vi "Full Code using SensorDAQ.vi"() -> ()   [LabVIEW 2012]
uses:
  <vilib>/Utility/file.llb/Write To Spreadsheet File (string).vi
  <vilib>/express/express arith-compare/Formula/XNode/ExpressFormulaBlockNode.xnode
panel:
  in  "?":bool
  out "Nitrogen Compounds \n(NOx)  ppm":dbl(graph)
  out "Chlorine Gas (Cl2)  ppm":dbl(graph)
  out "Ozone (O3) ppm":dbl(graph)
  out "Nitrogen Compounds \n(NOx)  ppm_percentage":dbl
  out "Chlorine Gas (Cl2)  ppm_percentage":dbl
  out "Ozone (O3) ppm_percentage":dbl
  out "Nitrogen Compounds \n(NOx)  ppm":dbl
  out "Chlorine Gas (Cl2)  ppm":dbl
  out "Ozone (O3) ppm":dbl
  in  "Ro for MQ131":dbl
  out "Methane (CH4)  ppm":dbl(graph)
  out "Carbon Monoxide (CO)  ppm":dbl(graph)
  out "Butane (LPG) ppm":dbl(graph)
  out "Methane (CH4)\nppm_percentage":dbl
  out "Carbon Monoxide (CO)  ppm_percentage":dbl
  out "Butane (LPG) ppm_percentage":dbl
  out "Methane (CH4)  ppm":dbl
  out "Carbon Monoxide (CO)  ppm":dbl
  out "Butane   (LPG) ppm":dbl
  in  "Ro for MQ9":dbl
  out "CH 3 PH":dbl caption="CH 3 Auto-ID"
  out "CH 2 Conductivity":dbl caption="CH 2 Auto-ID"
  out "CH 1 Temperature":dbl caption="CH 1 Auto-ID"
  in  "file path (use dialog)":path
  out "Raw Voltage MQ9 Gas Sensor":dbl
  out "Raw Voltage MQ131 Ozone Sensor":dbl
  # "Vernier Sensors"
  # "MQ9 Gas Sensor"
  # "MQ131 Ozone Sensor"
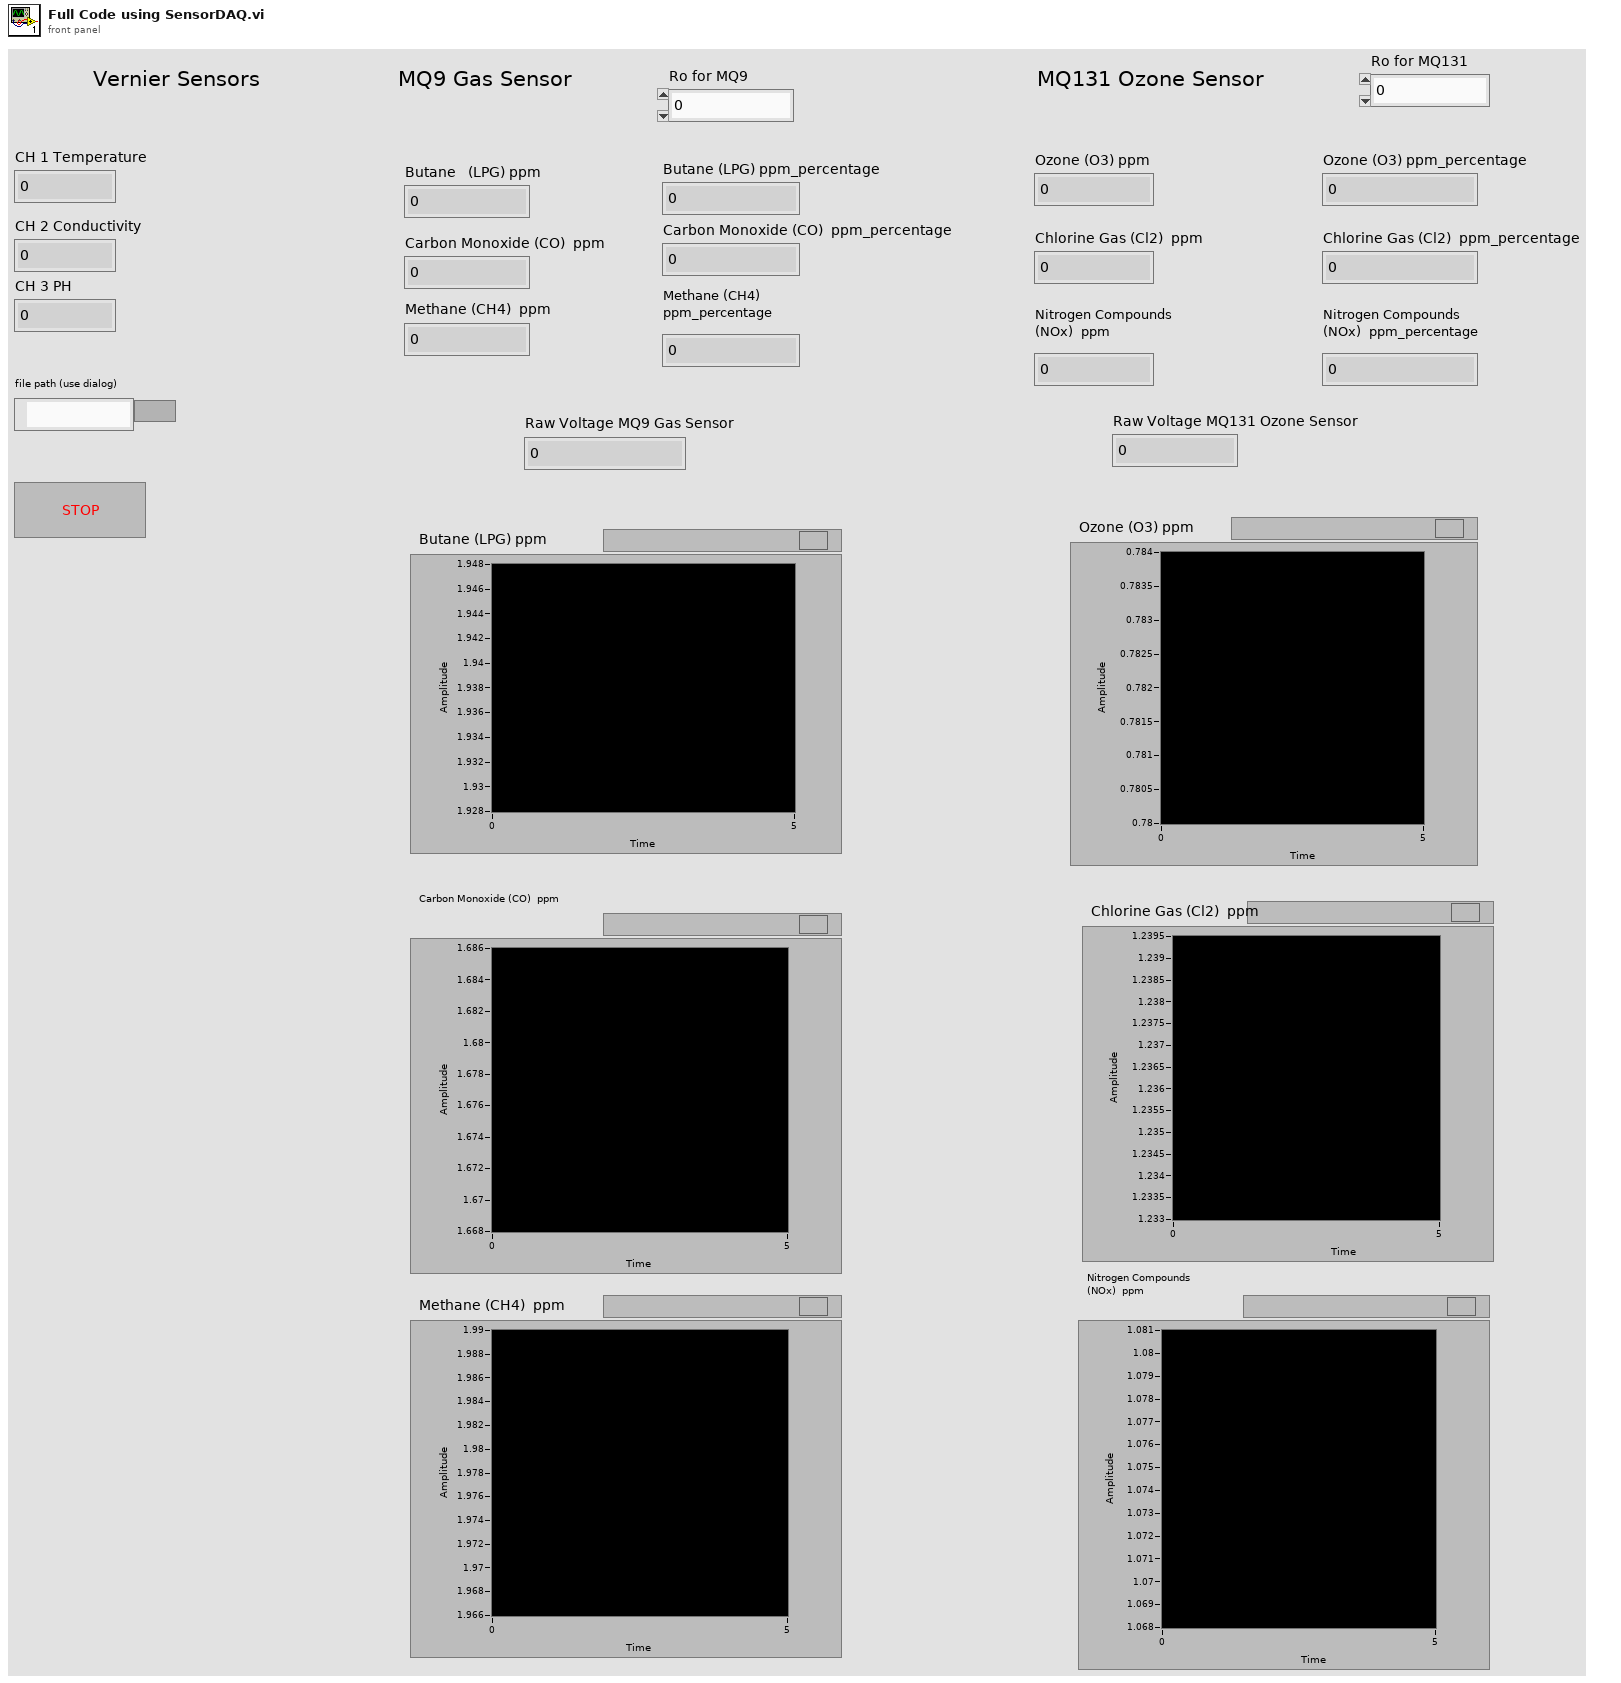
[diagram p1: front panel]
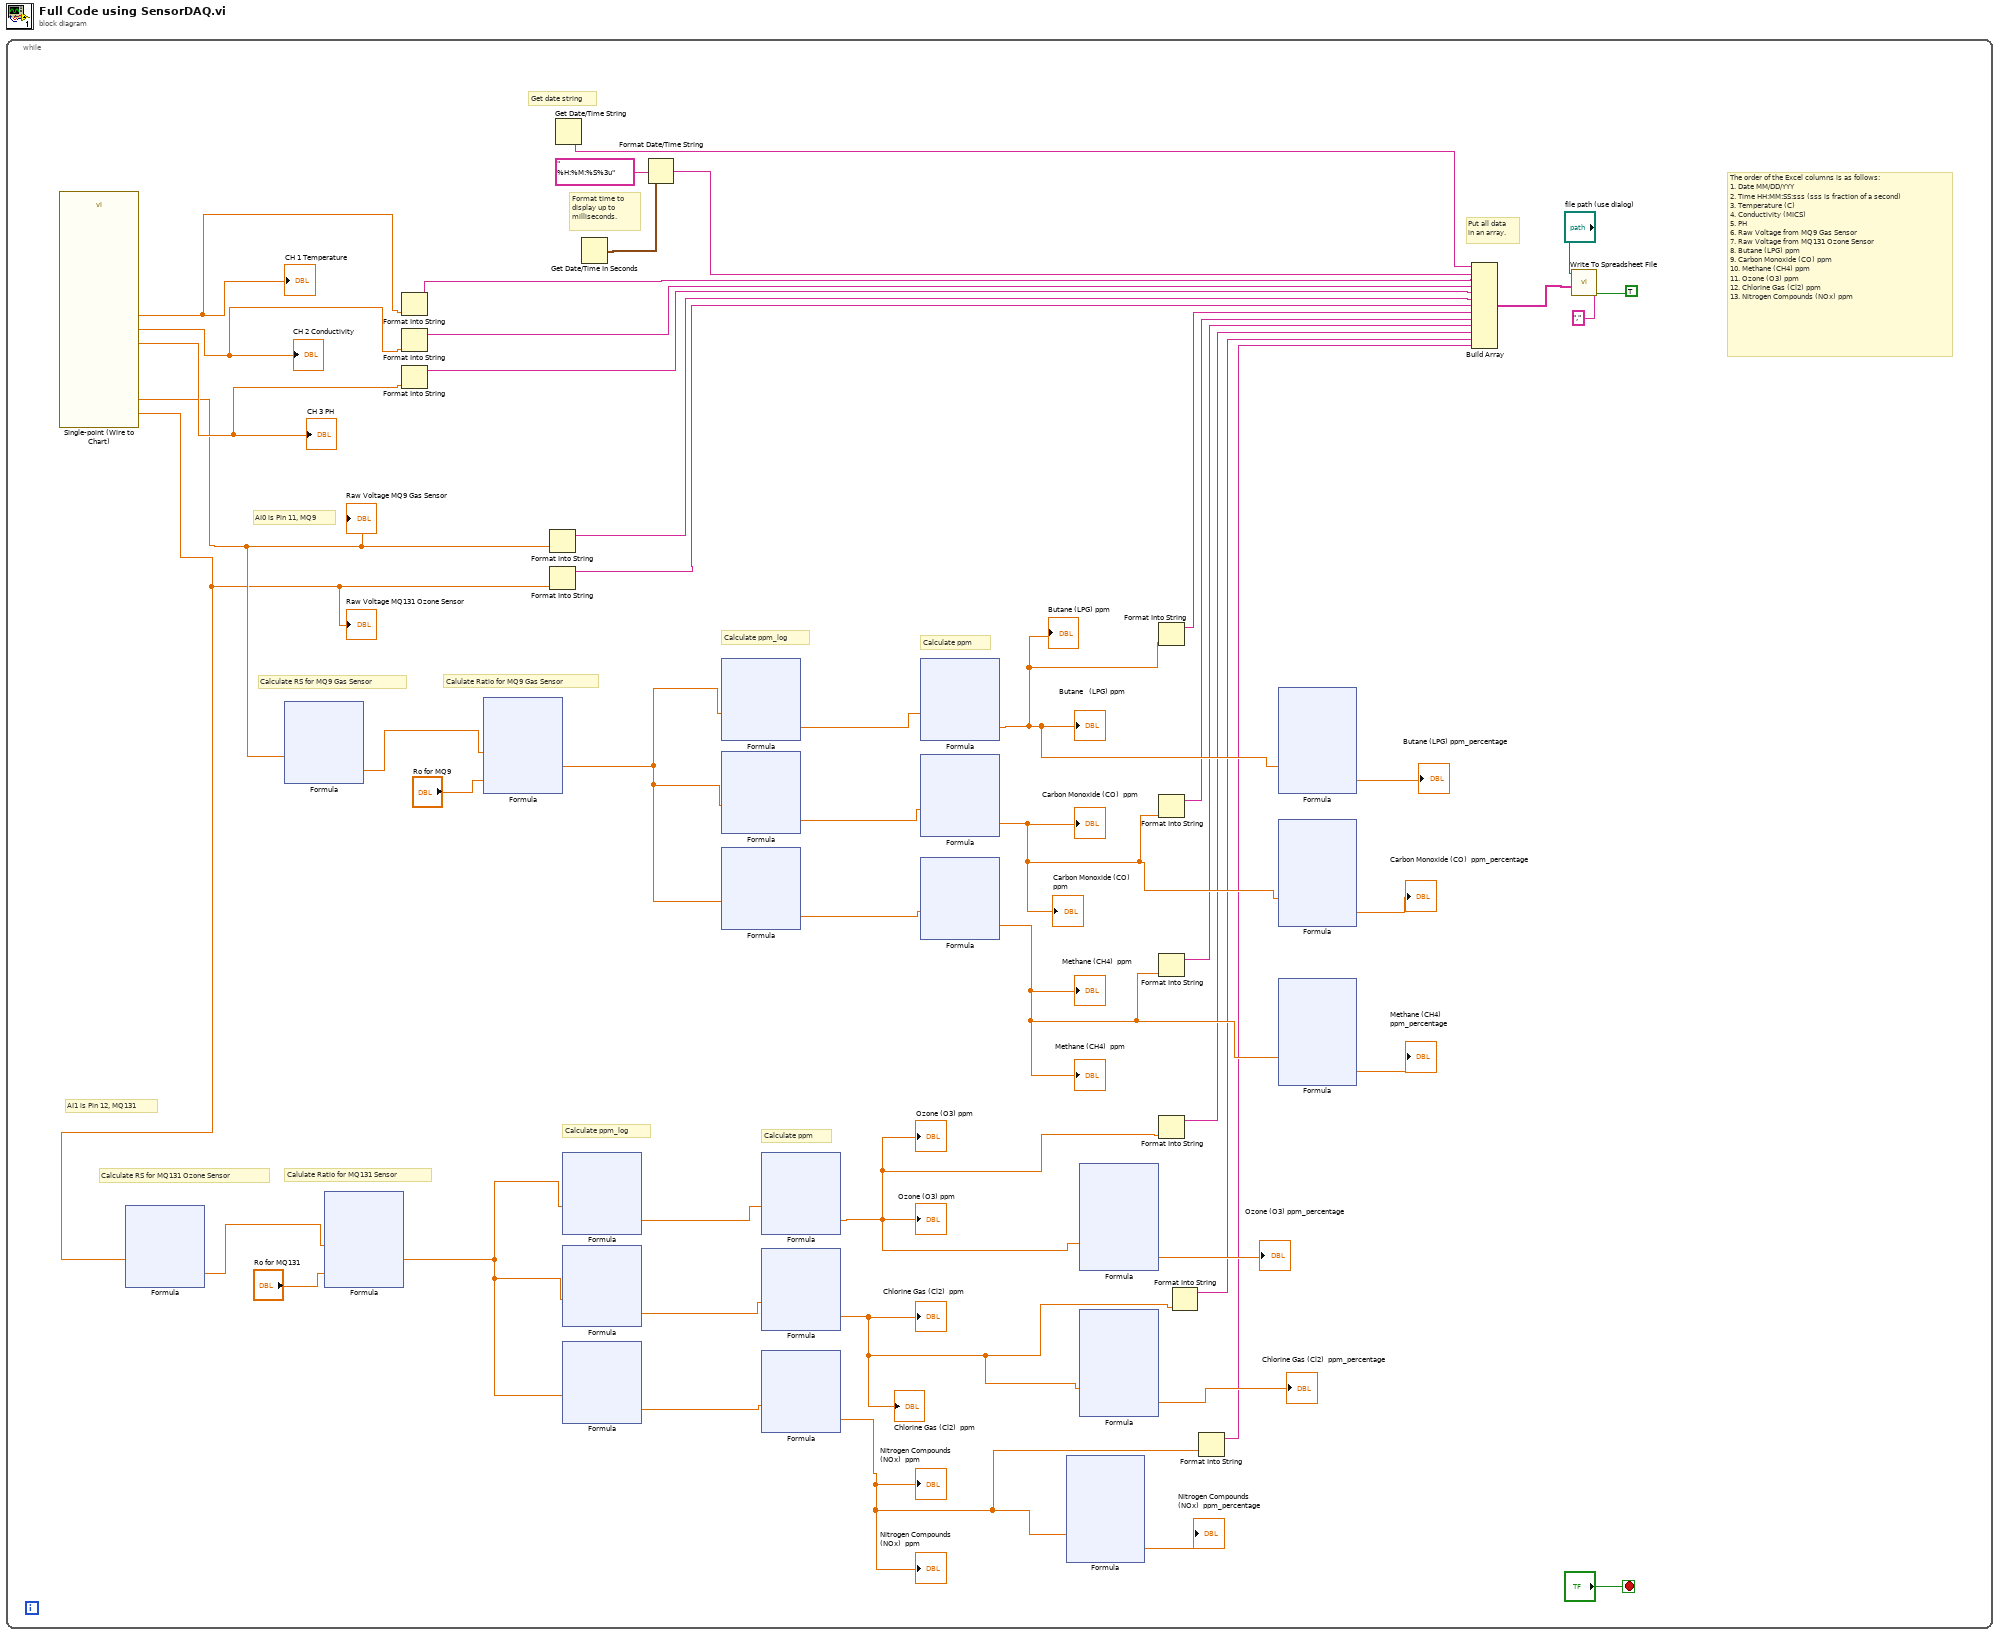
[diagram p0: block diagram]
diagram:
  n1 = while {
    stop <- "?" stop-if-true
    # "AI1 is Pin 12, MQ131"
    # "AI0 is Pin 11, MQ9"
    # "Calculate ppm"
    # "Calculate ppm_log"
    # "Calulate Ratio for MQ131 Sensor"
    # "Calculate RS for MQ131 Ozone Sensor"
    # "Calculate ppm"
    # "Calculate ppm_log"
    # "Calulate Ratio for MQ9 Gas Sensor"
    # "Calculate RS for MQ9 Gas Sensor"
    # "The order of the Excel columns is as follows:\n1. Date MM/DD/YYY\n2. Time HH:MM:SS:sss (sss is fraction of a second)\n3. Temperature (C)\n4. Conductivity (MICS)\n5. PH\n6. Raw Voltage from MQ9 Gas Sensor\n7. Raw Voltage from MQ131 Ozone Sensor\n8. Butane (LPG) ppm\n9. Carbon Monoxide (CO) ppm\n10. Methane (CH4) ppm\n11. Ozone (O3) ppm\n12. Chlorine Gas (Cl2) ppm\n13. Nitrogen Compounds (NOx) ppm"
    # "Put all data\nin an array."
    # "Format time to \ndisplay up to\nmilliseconds."
    # "Get date string"
    n2 = call "Single-point (Wire to Chart)"() -> ("Temp1 ºC"=w41:dbl, "CONDUCT2 (MICS)"=w40:dbl, "PH3"=w39:dbl, "AI0 pin 11 RSE"=w2:dbl, "AI1 pin 12 RSE"=w1:dbl)  [unwired: 12 in, 3 out]
    "Raw Voltage MQ9 Gas Sensor" <- w2
    "Raw Voltage MQ131 Ozone Sensor" <- w1
    "CH 1 Temperature" <- w41
    "CH 2 Conductivity" <- w40
    "CH 3 PH" <- w39
    n3 = xnode "Formula"("X1"=w1) -> ("Result"=w23:dbl)  [unwired: 1 in, 1 out]
    n4 = xnode "Formula"("X1"=w2) -> ("Result"=w32:dbl)  [unwired: 1 in, 1 out]
    n5 = xnode "Formula"("X1"=w23, "X2"="Ro for MQ131") -> ("Result"=w22:dbl)  [unwired: 1 in, 1 out]
    n6 = Format Into String(w41) -> (resulting string=w38:string)  [unwired: 3 in, 1 out]
    n7 = Format Into String(w40) -> (resulting string=w37:string)  [unwired: 3 in, 1 out]
    n8 = Format Into String(w39) -> (resulting string=w36:string)  [unwired: 3 in, 1 out]
    n9 = xnode "Formula"("X1"=w32, "X2"="Ro for MQ9") -> ("Result"=w31:dbl)  [unwired: 1 in, 1 out]
    n10 = Format Into String(w2) -> (resulting string=w35:string)  [unwired: 3 in, 1 out]
    n11 = Format Into String(w1) -> (resulting string=w34:string)  [unwired: 3 in, 1 out]
    n12 = Get Date/Time String() -> (date string=w45:string)  [unwired: 3 in, 1 out]
    n13 = xnode "Formula"("X1"=w22) -> ("Result"=w21:dbl)  [unwired: 1 in, 1 out]
    n14 = xnode "Formula"("X1"=w22) -> ("Result"=w20:dbl)  [unwired: 1 in, 1 out]
    n15 = xnode "Formula"("X1"=w22) -> ("Result"=w19:dbl)  [unwired: 1 in, 1 out]
    n16 = Get Date/Time In Seconds() -> (seconds since 1Jan1904=w43:timestamp)
    n17 = Format Date/Time String(time format string (%c)="            %H:%M:%S%3u", seconds (now)=w43) -> (date/time string=w44:string)  [unwired: 1 in]
    n18 = xnode "Formula"("X1"=w31) -> ("Result"=w30:dbl)  [unwired: 1 in, 1 out]
    n19 = xnode "Formula"("X1"=w31) -> ("Result"=w29:dbl)  [unwired: 1 in, 1 out]
    n20 = xnode "Formula"("X1"=w31) -> ("Result"=w28:dbl)  [unwired: 1 in, 1 out]
    n21 = xnode "Formula"("X1"=w21) -> ("Result"=w14:dbl)  [unwired: 1 in, 1 out]
    "Ozone (O3) ppm" <- w14
    "Ozone (O3) ppm" <- w14
    n22 = xnode "Formula"("X1"=w20) -> ("Result"=w13:dbl)  [unwired: 1 in, 1 out]
    "Chlorine Gas (Cl2)  ppm" <- w13
    "Chlorine Gas (Cl2)  ppm" <- w13
    n23 = xnode "Formula"("X1"=w19) -> ("Result"=w12:dbl)  [unwired: 1 in, 1 out]
    "Nitrogen Compounds \n(NOx)  ppm" <- w12
    "Nitrogen Compounds \n(NOx)  ppm" <- w12
    n24 = xnode "Formula"("X1"=w30) -> ("Result"=w11:dbl)  [unwired: 1 in, 1 out]
    "Butane   (LPG) ppm" <- w11
    "Butane (LPG) ppm" <- w11
    n25 = xnode "Formula"("X1"=w29) -> ("Result"=w10:dbl)  [unwired: 1 in, 1 out]
    "Carbon Monoxide (CO)  ppm" <- w10
    "Carbon Monoxide (CO)  ppm" <- w10
    n26 = xnode "Formula"("X1"=w28) -> ("Result"=w9:dbl)  [unwired: 1 in, 1 out]
    "Methane (CH4)  ppm" <- w9
    "Methane (CH4)  ppm" <- w9
    n27 = xnode "Formula"("X1"=w12) -> ("Result"=→"Nitrogen Compounds \n(NOx)  ppm_percentage":dbl)  [unwired: 1 in, 1 out]
    n28 = xnode "Formula"("X1"=w14) -> ("Result"=→"Ozone (O3) ppm_percentage":dbl)  [unwired: 1 in, 1 out]
    n29 = xnode "Formula"("X1"=w13) -> ("Result"=→"Chlorine Gas (Cl2)  ppm_percentage":dbl)  [unwired: 1 in, 1 out]
    n30 = Format Into String(w11) -> (resulting string=w8:string)  [unwired: 3 in, 1 out]
    n31 = Format Into String(w10) -> (resulting string=w7:string)  [unwired: 3 in, 1 out]
    n32 = Format Into String(w9) -> (resulting string=w6:string)  [unwired: 3 in, 1 out]
    n33 = Format Into String(w14) -> (resulting string=w5:string)  [unwired: 3 in, 1 out]
    n34 = Format Into String(w13) -> (resulting string=w4:string)  [unwired: 3 in, 1 out]
    n35 = Format Into String(w12) -> (resulting string=w3:string)  [unwired: 3 in, 1 out]
    n36 = xnode "Formula"("X1"=w11) -> ("Result"=→"Butane (LPG) ppm_percentage":dbl)  [unwired: 1 in, 1 out]
    n37 = xnode "Formula"("X1"=w10) -> ("Result"=→"Carbon Monoxide (CO)  ppm_percentage":dbl)  [unwired: 1 in, 1 out]
    n38 = xnode "Formula"("X1"=w9) -> ("Result"=→"Methane (CH4)\nppm_percentage":dbl)  [unwired: 1 in, 1 out]
    n39 = Build Array(w45, w44, w38, w37, w36, w35, w34, w8, w7, w6, w5, w4, w3) -> (w42:string[])
    n40 = call-poly <vilib>:"Write To Spreadsheet File.vi"("delimiter (\\t)"="," ("delimiter (\\t)"), "append to file? (new file:F)"=TRUE, "1D data"=w42, "file path (dialog if empty)"="file path (use dialog)") -> ()  [unwired: 4 in, 1 out]
  }
